vi "current monitor2.vi"() -> ()   [LabVIEW 2010]
uses:
  <vilib>/Utility/file.llb/Write To Spreadsheet File (DBL).vi
  <userlib>/Nanonis Prog Interface V5/Nanonis Prog Interface.lvlib
panel:
  in  "Convert to nm/s?":bool caption="Spectrum Analyzer 2"
  out "Spectrum Analyzer 2":cluster{"f0":dbl, "df":dbl, "values":dbl[]}(graph)
  in  "Spectrum Analyzer2":bool caption="Spectrum Analyzer 2"
  out "error out":errorcluster
  in  "Path":path
  out "Spectrum Analyzer":cluster{"f0":dbl, "df":dbl, "values":dbl[]}(graph)
  out "Current (A)":sgl format="%#_6p"
  out "Current":cluster{"Current (A)":dbl, dbl}[](graph)
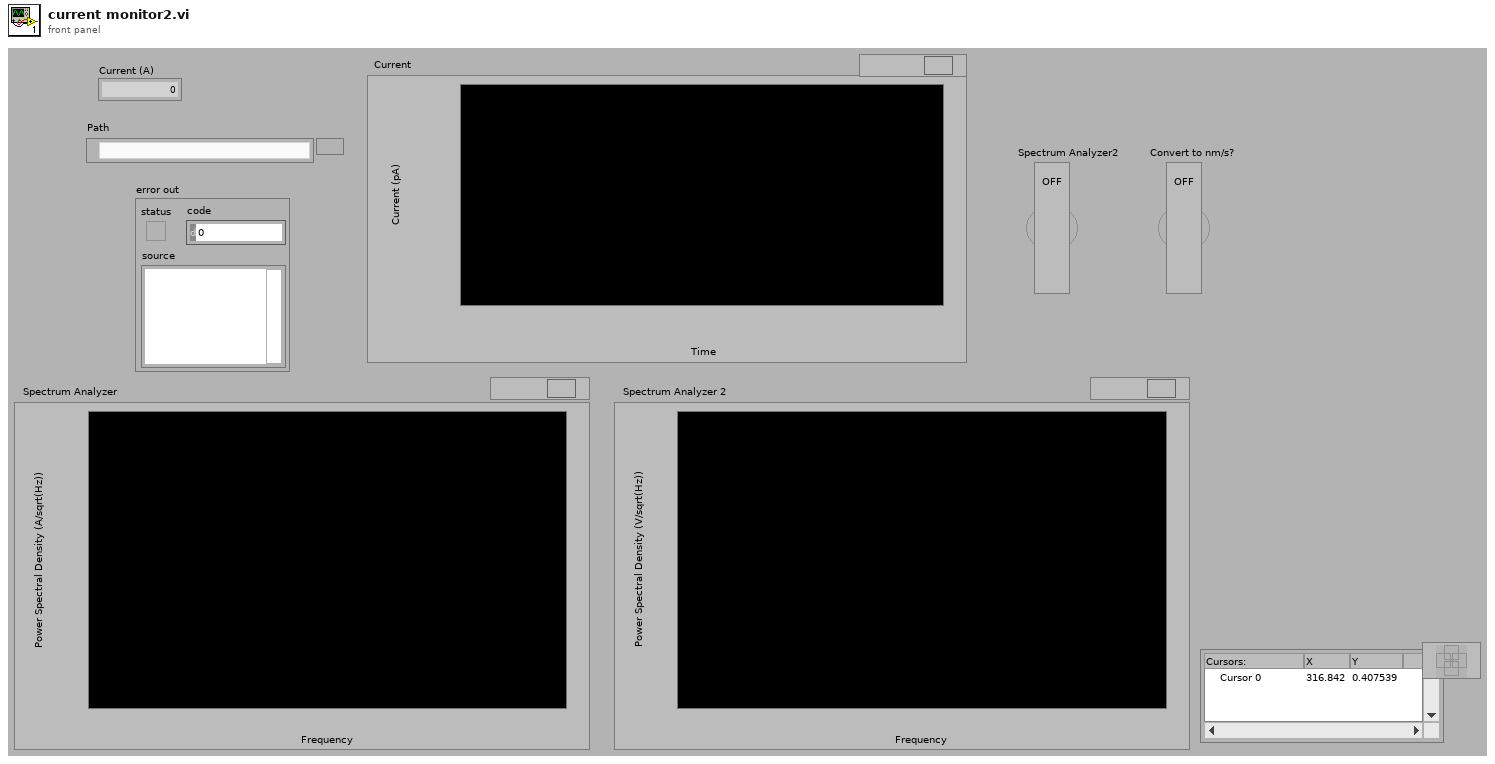
[diagram p1: front panel]
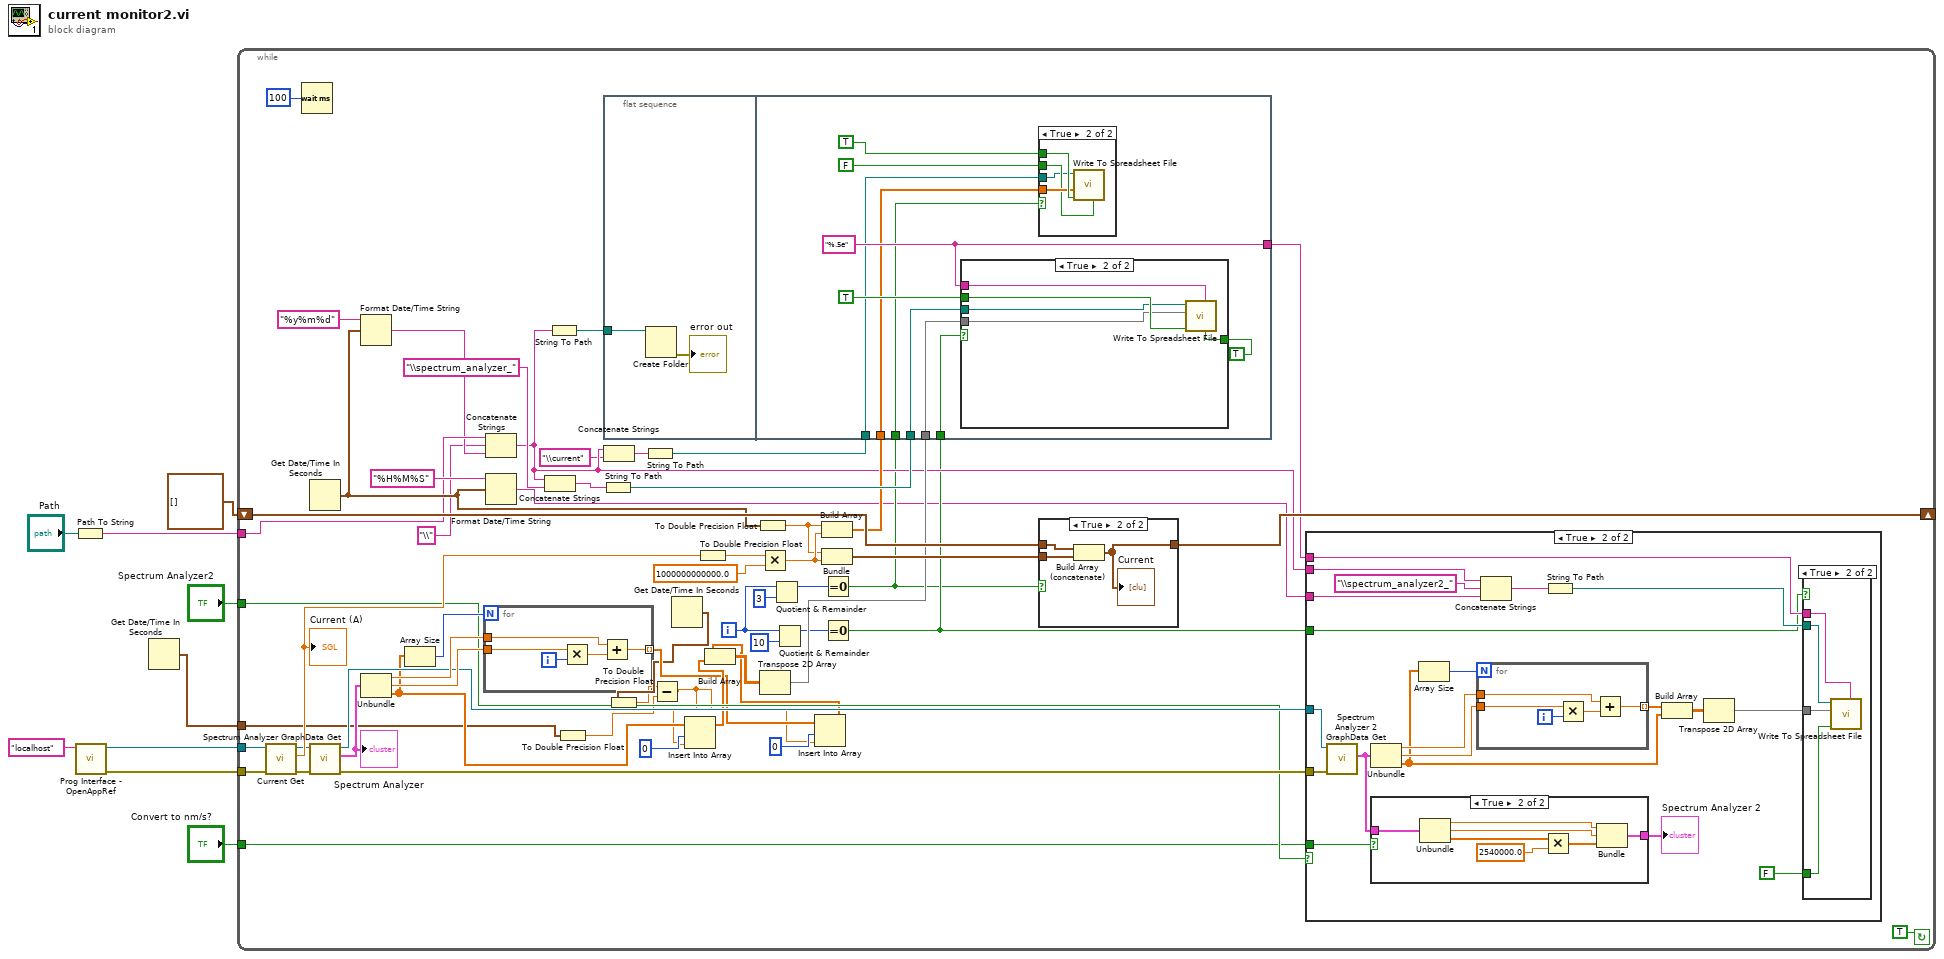
[diagram p0: block diagram]
diagram:
  n1 = Path To String(path="Path") -> (string=w4:string)
  n2 = call <userlib>:"Prog Interface - OpenAppRef.vi"("Machine name (local machine IP)"="localhost" ("machine name (localhost)")) -> ("Error out"=w8:errorcluster, "Application reference"=w9:refnum<vi>)  [unwired: 5 in]
  n3 = Get Date/Time In Seconds() -> (seconds since 1Jan1904=w1:timestamp)
  n4 = while {
    tunnel: w9 -> [w67]
    tunnel: w8 -> [w66]
    shift-right: [w63] -> _
    shift-left: cluster{dbl, dbl}[] [] -> [w64]
    tunnel: w4 -> [w51]
    tunnel: "Spectrum Analyzer2" -> [w38]
    tunnel: "Convert to nm/s?" -> [w36]
    tunnel: w1 -> [w10]
    i -> [w23]
    stop <- TRUE continue-if-true
    n5 = call <userlib>:"Current Get.vi"("Error in (no error)"=w66, "Application ref in"=w67) -> ("Error out"=w58:errorcluster, "Current (A)"=w62:sgl, "Application ref out"=w59:refnum<vi>)  [unwired: 5 in]
    "Current (A)" <- w62
    n6 = Wait (ms)(milliseconds to wait=u32 100) -> ()  [unwired: 1 out]
    n7 = Get Date/Time In Seconds() -> (seconds since 1Jan1904=w52:timestamp)
    n8 = call <userlib>:"Spectrum Analyzer GraphData Get.vi"("Error in (no error)"=w58, "Application ref in"=w59) -> ("Error out"=w39:errorcluster, "FFT data"=w56:cluster{"f0":dbl, "df":dbl, "values":dbl[]}, "Application ref out"=w40:refnum<vi>)  [unwired: 7 in]
    "Spectrum Analyzer" <- w56
    n9 = Format Date/Time String(time format string (%c)="%y%m%d", seconds (now)=w52) -> (date/time string=w49:string)  [unwired: 1 in]
    n10 = Unbundle(w56) -> ("f0"=w44:dbl, "df"=w43:dbl, "values"=w19:dbl[])
    n11 = Array Size(array=w19) -> (size(s)=w45:i32)
    n12 = for {
      N: w45 -> [_]
      tunnel: w44 -> [w114]
      tunnel: w43 -> [w111]
      tunnel: [w110] -> w16 mode=indexing
      i -> [w112]
      n13 = Multiply(x=w111, y=w112) -> (x*y=w113:dbl)
      n14 = Add(x=w114, y=w113) -> (x+y=w110:dbl)
    }
    n15 = Concatenate Strings(w51, "\\" ("string"), w49) -> (w34:string)
    n16 = Format Date/Time String(time format string (%c)="%H%M%S", seconds (now)=w52) -> (date/time string=w21:string)  [unwired: 1 in]
    n17 = Concatenate Strings(w34, "\\spectrum_analyzer_" ("string")) -> (w46:string)
    n18 = String To Path(string=w34) -> (path=w50:path)
    n19 = To Double Precision Float(number=w10) -> (double precision float=w11:dbl)
    n20 = String To Path(string=w46) -> (path=w54:path)
    n21 = flat-sequence {
      tunnel: w50 -> [w116]
      tunnel: w54 -> [w120]
      tunnel: w41 -> [w121]
      tunnel: [w126] -> w37
      tunnel: w35 -> [w124]
      tunnel: w31 -> [w122]
      tunnel: w26 -> [w119]
      tunnel: w22 -> [w118]
      frame #0 {
        n22 = Create Folder(path (use dialog)=w116) -> (error out=→"error out":errorcluster)  [unwired: 2 in, 2 out]
      }
      frame #1 {
        w126 = "%.5e" ("format (%.3f)")
        n23 = case shown="True" w119 {
          tunnel: TRUE ("append to file? (new file:F)") -> [_ w136]
          tunnel: w126 -> [_ w135]
          tunnel: w121 -> [_ w134]
          tunnel: w120 -> [_ w133]
          tunnel: TRUE -> [_ w132]
          frame False {
          }
          frame True {
            n24 = call-poly <vilib>:"Write To Spreadsheet File.vi"("transpose? (no:F)"=w132, "format (%.3f)"=w135, "append to file? (new file:F)"=w136, "2D data"=w134, "file path (dialog if empty)"=w133) -> ()  [unwired: 3 in, 1 out]
          }
        }
        n25 = case shown="True" w118 {
          tunnel: TRUE ("append to file? (new file:F)") -> [_ w131]
          tunnel: w124 -> [_ w130]
          tunnel: FALSE ("transpose? (no:F)") -> [_ w129]
          tunnel: w122 -> [_ w128]
          frame False {
          }
          frame True {
            n26 = call-poly <vilib>:"Write To Spreadsheet File.vi"("transpose? (no:F)"=w129, "append to file? (new file:F)"=w131, "1D data"=w130, "file path (dialog if empty)"=w128) -> ()  [unwired: 4 in, 1 out]
          }
        }
      }
    }
    n27 = Concatenate Strings(w34, "\\current" ("string")) -> (w32:string)
    n28 = String To Path(string=w32) -> (path=w31:path)
    n29 = Get Date/Time In Seconds() -> (seconds since 1Jan1904=w13:timestamp)
    n30 = To Double Precision Float(number=w13) -> (double precision float=w12:dbl)
    n31 = Subtract(x=w12, y=w11) -> (x-y=w14:dbl)
    n32 = Insert Into Array(array=w19, index=0, new element=w14) -> (w18:dbl[])
    n33 = To Double Precision Float(number=w62) -> (double precision float=w61:dbl)
    n34 = To Double Precision Float(number=w52) -> (double precision float=w29:dbl)
    n35 = Multiply(x=w61, y=1000000000000.0) -> (x*y=w30:dbl)
    n36 = Quotient & Remainder(x=w23, y=3) -> (x-y*floor(x/y)=w24:i32)  [unwired: 1 out]
    n37 = Quotient & Remainder(x=w23, y=10) -> (x-y*floor(x/y)=w27:i32)  [unwired: 1 out]
    n38 = Insert Into Array(array=w16, index=0, new element=w14) -> (w15:dbl[])
    n39 = Build Array(w15, w18) -> (w42:dbl[][])
    n40 = Transpose 2D Array(2D array=w42) -> (transposed array=w41:dbl[][])
    n41 = Build Array(w29, w30) -> (w35:dbl[])
    n42 = Bundle(w29, w30) -> (w65:cluster{dbl, dbl})  [unwired: 1 in]
    n43 = Equal To 0?(x=w24) -> (x = 0?=w22:bool)
    n44 = Equal To 0?(x=w27) -> (x = 0?=w26:bool)
    n45 = case shown="True" w22 {
      tunnel: w65 -> [_ w72]
      tunnel: w64 -> [w69 w71]
      tunnel: [w69 w70] -> w63
      frame False {
      }
      frame True {
        n46 = Build Array (concatenate)(w71, w72) -> (w70:cluster{dbl, dbl}[])
        "Current" <- w70
      }
    }
    n47 = case shown="True" w38 {
      tunnel: w40 -> [_ w92]
      tunnel: w39 -> [_ w91]
      tunnel: w34 -> [_ w82]
      tunnel: w21 -> [_ w81]
      tunnel: w37 -> [_ w77]
      tunnel: w36 -> [_ w74]
      tunnel: w26 -> [_ w73]
      frame False {
      }
      frame True {
        n48 = call <userlib>:"Spectrum Analyzer 2 GraphData Get.vi"("Error in (no error)"=w91, "Application ref in"=w92) -> ("FFT data"=w76:cluster{"f0":dbl, "df":dbl, "values":dbl[]})  [unwired: 7 in, 2 out]
        n49 = Unbundle(w76) -> ("f0"=w89:dbl, "df"=w88:dbl, "values"=w86:dbl[])
        n50 = case shown="True" w74 {
          tunnel: w76 -> [w97 w104]
          tunnel: [w97 w103] -> w75
          frame False {
          }
          frame True {
            n51 = Unbundle(w104) -> ("f0"=w102:dbl, "df"=w101:dbl, "values"=w100:dbl[])
            n52 = Multiply(x=w100, y=2540000.0) -> (x*y=w99:dbl[])
            n53 = Bundle("f0"=w102, "df"=w101, w99) -> (w103:cluster{"f0":dbl, "df":dbl, dbl[]})  [unwired: 1 in]
          }
        }
        "Spectrum Analyzer 2" <- w75
        n54 = Array Size(array=w86) -> (size(s)=w90:i32)
        n55 = for {
          N: w90 -> [_]
          tunnel: w89 -> [w109]
          tunnel: w88 -> [w106]
          tunnel: [w105] -> w85 mode=indexing
          i -> [w107]
          n56 = Multiply(x=w106, y=w107) -> (x*y=w108:dbl)
          n57 = Add(x=w109, y=w108) -> (x+y=w105:dbl)
        }
        n58 = Concatenate Strings(w82, "\\spectrum_analyzer2_" ("string"), w81) -> (w78:string)
        n59 = String To Path(string=w78) -> (path=w79:path)
        n60 = Build Array(w85, w86) -> (w87:dbl[][])
        n61 = Transpose 2D Array(2D array=w87) -> (transposed array=w83:dbl[][])
        n62 = case shown="True" w73 {
          tunnel: FALSE ("append to file? (new file:F)") -> [_ w96]
          tunnel: w83 -> [_ w95]
          tunnel: w79 -> [_ w94]
          tunnel: w77 -> [_ w93]
          frame False {
          }
          frame True {
            n63 = call-poly <vilib>:"Write To Spreadsheet File.vi"("format (%.3f)"=w93, "append to file? (new file:F)"=w96, "2D data"=w95, "file path (dialog if empty)"=w94) -> ()  [unwired: 4 in, 1 out]
          }
        }
      }
    }
  }
